vi "parse user credentials.vi"(7 "ENV":T1, 8 "error in (no error)":errorcluster, 9 "Logout? (f)":bool, 10 "Post Data (\"\")":string, 11 "Connection Refnum":T2) -> (0 "error out":errorcluster, 1 "Login?":bool, 2 "Response Header":string, 3 "dup Connection Refnum":T2, 4 "attempts":i32, 5 "updated ENV":T1, 6 "User":T3)   [LabVIEW 2011]
uses:
  ITK EXT/utils/keyedarr.llb/Keyed Array.ctl
  server/database/Users/User Record.ctl
  Summitek EXT/ODBC/SQL Controls/Connection Refnum.ctl
  ITK EXT/utils/strutil.llb/Case Matching.ctl
  server/server lib/Spartan CONFIG Global.vi
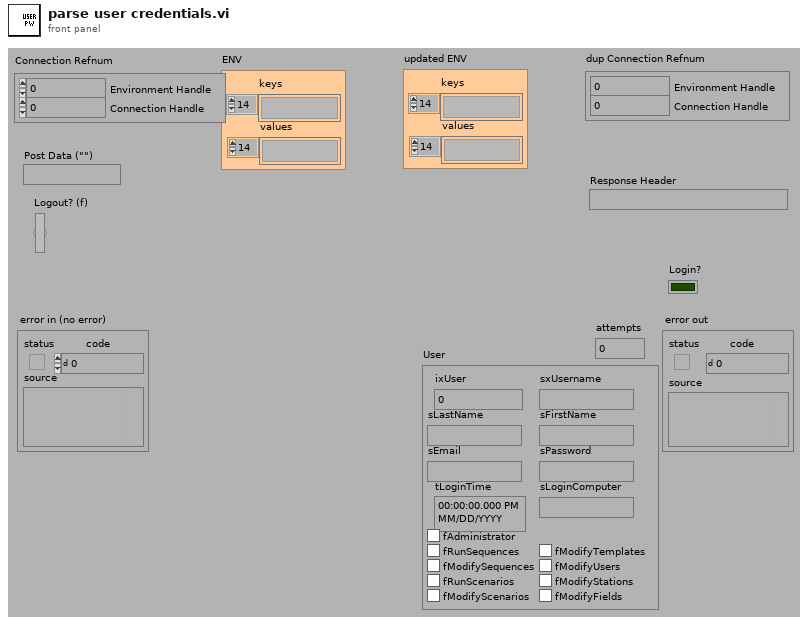
[diagram p1: front panel]
types:
  T1 = typedef "Keyed Array.ctl" = cluster{"keys":string[], "values":string[]}
  T2 = typedef "Connection Refnum.ctl" = cluster{"Environment Handle":i32, "Connection Handle":i32}
  T3 = typedef "User Record.ctl" = cluster{"ixUser":i32, "sxUsername":string, "sLastName":string, "sFirstName":string, "sEmail":string, "sPassword":string, "tLoginTime":timestamp, "sLoginComputer":string, "fAdministrator":bool, "fRunSequences":bool, "fModifySequences":bool, "fRunScenarios":bool, "fModifyScenarios":bool, "fModifyTemplates":bool, "fModifyUsers":bool, "fModifyStations":bool, "fModifyFields":bool}
  T4 = typedef "Case Matching.ctl" = enum16{"a != A", "a == A", "system"}
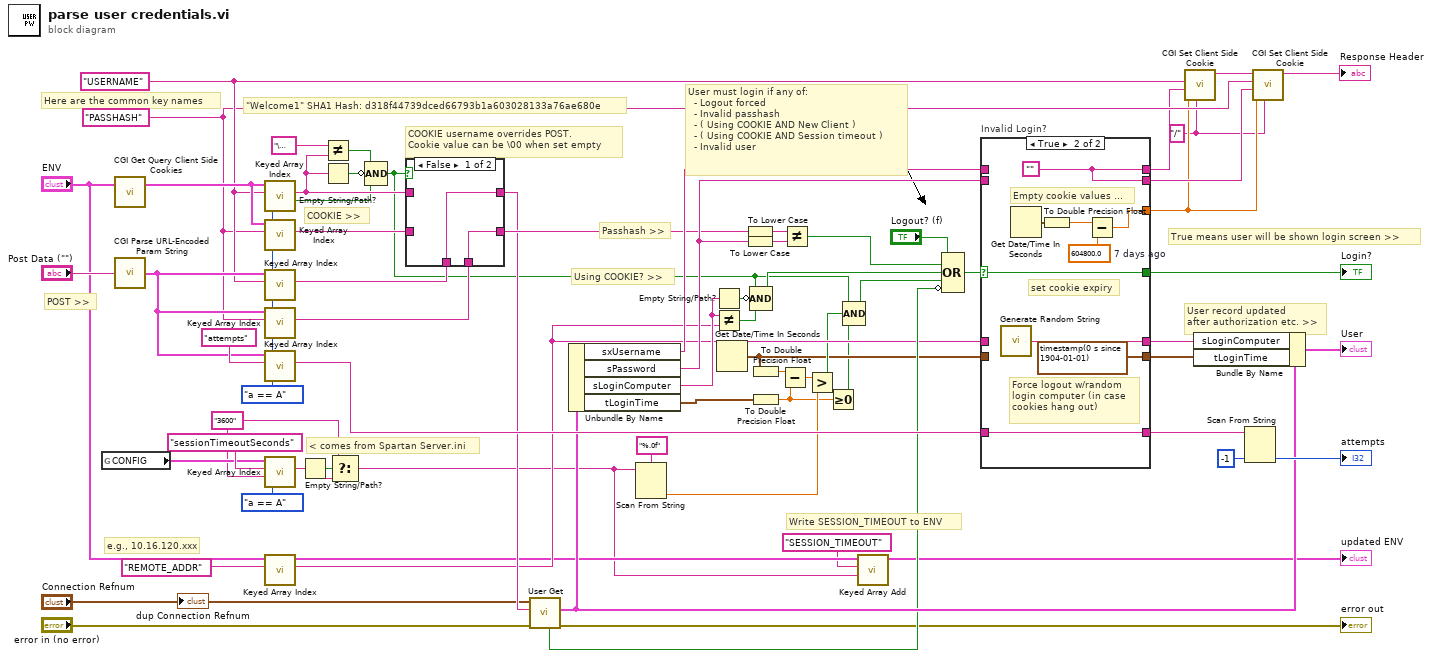
[diagram p0: block diagram]
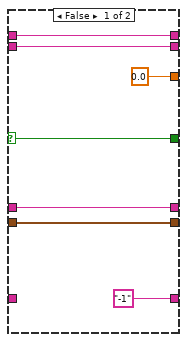
[diagram p3: hidden frame]
diagram:
  w3 = "3600" ("default value")
  w24 = "/"
  w16 = Case_Matching."a == A" ("case matching (sensitive)")
  w41 = "PASSHASH"
  w42 = "USERNAME"
  # "< comes from Spartan Server.ini"
  # "Write SESSION_TIMEOUT to ENV"
  # "Using COOKIE? >>"
  # "\"Welcome1\" SHA1 Hash: d318f44739dced66793b1a603028133a76ae680e"
  # "User record updated\nafter authorization etc. >>"
  # "COOKIE >>"
  # "POST >>"
  # "Passhash >>"
  # "Here are the common key names"
  # "COOKIE username overrides POST.\nCookie value can be \\00 when set empty"
  # "User must login if any of:\n  - Logout forced\n  - Invalid passhash\n  - ( Using COOKIE AND New Client )\n  - ( Using COOKIE AND Session timeout )\n  - Invalid user"
  # "True means user will be shown login screen >>"
  # "e.g., 10.16.120.xxx"
  n1 = global read "Spartan CONFIG Global.vi" "CONFIG"() -> (w13:T1)
  n2 = call "CGI Get Query Client Side Cookies.vi"("env"="ENV") -> ("client cookies"=w67:T1)  [unwired: 2 out]
  n3 = call "CGI Parse URL-Encoded Param String.vi"("url-encoded param string"="Post Data (\"\")") -> ("params"=w68:T1)
  n4 = call "Keyed Array Index.vi"("case matching (sensitive)"=w16, "key"=w42, "array in"=w67) -> ("valid key"=w31:bool, "value"=w32:string)  [unwired: 1 in, 2 out]
  n5 = call "Keyed Array Index.vi"("case matching (sensitive)"=w16, "key"=w41, "array in"=w67) -> ("value"=w40:string)  [unwired: 1 in, 3 out]
  n6 = call "Keyed Array Index.vi"("case matching (sensitive)"=w16, "key"=w42, "array in"=w68) -> ("value"=w37:string)  [unwired: 1 in, 3 out]
  n7 = call "Keyed Array Index.vi"("case matching (sensitive)"=w16, "key"=w41, "array in"=w68) -> ("value"=w36:string)  [unwired: 1 in, 3 out]
  n8 = call "Keyed Array Index.vi"("case matching (sensitive)"=w16, "key"="attempts", "array in"=w68) -> ("value"=w69:string)  [unwired: 1 in, 3 out]
  n9 = call "Keyed Array Index.vi"("case matching (sensitive)"=Case_Matching."a == A", "default value"=w3, "key"="sessionTimeoutSeconds", "array in"=w13) -> ("value"=w1:string)  [unwired: 3 out]
  n10 = call "Keyed Array Index.vi"("key"="REMOTE_ADDR" ("Spartan User Credential Cookie"), "array in"="ENV") -> ("value"=w28:string, "duplicate array"=w12:T1)  [unwired: 2 in, 2 out]
  n11 = Empty String/Path?(string/path=w1) -> (empty?=w4:bool)
  n12 = Not Equal?(x="\u0000" ("value"), y=w32) -> (x != y?=w33:bool)
  n13 = Empty String/Path?(string/path=w32) -> (empty?=w35:bool)
  n14 = Select(t=w3, s=w4, f=w1) -> (s? t:f=w2:string)
  n15 = Compound Arithmetic op=AND(w33, invert w35, w31) -> (w21:bool)
  n16 = case shown="False" w21 {
    tunnel: w32 -> [_ w74]
    tunnel: [w72 w75] -> w39
    tunnel: w40 -> [_ w75]
    tunnel: [w73 w74] -> w38
    tunnel: w37 -> [w73 _]
    tunnel: w36 -> [w72 _]
    frame False {
    }
    frame True {
    }
  }
  n17 = call "User Get.vi"("error in (no error)"="error in (no error)", "sxUsername (\"\")"=w38, "Connection Refnum"="Connection Refnum") -> ("error out"=→"error out":errorcluster, "User"=w60:T3, "Data Present?"=w57:bool)  [unwired: 6 out]
  n18 = Unbundle By Name(w60) -> ("sxUsername"=w46:string, "sPassword"=w45:string, "sLoginComputer"=w44:string, "tLoginTime"=w23:timestamp)
  n19 = Scan From String(format string="%.0f", input string=w2) -> (output 1=w8:dbl)  [unwired: 2 in, 4 out]
  n20 = Empty String/Path?(string/path=w44) -> (empty?=w7:bool)
  n21 = Not Equal?(x=w44, y=w28) -> (x != y?=w43:bool)
  n22 = Get Date/Time In Seconds() -> (seconds since 1Jan1904=w18:timestamp)
  n23 = To Lower Case(string=w39) -> (all lower case string=w52:string)
  n24 = To Lower Case(string=w45) -> (all lower case string=w51:string)
  n25 = Compound Arithmetic op=AND(w21, invert w7, w43) -> (w50:bool)
  n26 = To Double Precision Float(number=w18) -> (double precision float=w19:dbl)
  n27 = To Double Precision Float(number=w23) -> (double precision float=w6:dbl)
  n28 = Subtract(x=w19, y=w6) -> (x-y=w49:dbl)
  n29 = Not Equal?(x=w52, y=w51) -> (x != y?=w53:bool)
  n30 = Greater?(x=w49, y=w8) -> (0:w20:bool)
  n31 = Greater Or Equal To 0?(x=w6) -> (x >= 0?=w5:bool)
  n32 = Compound Arithmetic op=AND(w21, w20, w5) -> (w22:bool)
  n33 = call "Keyed Array Add.vi"("value"=w2, "key"="SESSION_TIMEOUT", "array in"=w12) -> ("array out"=→"updated ENV":T1)  [unwired: 1 in, 3 out]
  n34 = Compound Arithmetic op=OR("Logout? (f)", w53, w50, w22, invert w57) -> (w48:bool)
  n35 = case "Invalid Login?" shown="True" w48 {
    selector: w48 -> [w81 w91]
    tunnel: ["-1" w89] -> w61
    tunnel: w69 -> [_ w89]
    tunnel: [w81 w91] -> w64
    tunnel: [w79 w88] -> w29
    tunnel: [w80 timestamp(0 s since 1904-01-01) ("tLoginTime")] -> w59
    tunnel: [w78 w83] -> w54
    tunnel: w18 -> [w80 _]
    tunnel: w46 -> [w79 _]
    tunnel: w45 -> [w77 _]
    tunnel: w28 -> [w78 _]
    tunnel: [w77 w88] -> w30
    tunnel: [0.0 ("expires (default)") w84] -> w25
    frame False {
    }
    frame True {
      w85 = 604800.0  # 7 days ago
      w88 = ""
      # "Force logout w/random\nlogin computer (in case\ncookies hang out)"
      # "set cookie expiry"
      # "Empty cookie values ..."
      n36 = call "Generate Random String.vi"() -> ("Output String"=w83:string)  [unwired: 1 in, 4 out]
      n37 = Get Date/Time In Seconds() -> (seconds since 1Jan1904=w87:timestamp)
      n38 = To Double Precision Float(number=w87) -> (double precision float=w86:dbl)
      n39 = Subtract(x=w86, y=w85) -> (x-y=w84:dbl)
    }
  }
  "Login?" <- w64
  n40 = call "CGI Set Client Side Cookie.vi"("path (\"\")"=w24, "expires (default)"=w25, "cookie value"=w29, "cookie name"=w42) -> ("header out"=w56:string)  [unwired: 1 in, 6 out]
  n41 = Bundle By Name(cluster=w60, "sLoginComputer"=w54, "tLoginTime"=w59) -> (→"User":T3)
  n42 = Scan From String(input string=w61, default 1=-1 ("default value 1")) -> (output 1=→"attempts":i32)  [unwired: 3 in, 3 out]
  n43 = call "CGI Set Client Side Cookie.vi"("path (\"\")"=w24, "expires (default)"=w25, "cookie value"=w30, "cookie name"=w41, "header in"=w56) -> ("header out"=→"Response Header":string)  [unwired: 6 out]
  "dup Connection Refnum" <- "Connection Refnum"
